vi "add points 2.0.vi"(10 "Spacing":dbl=1.0, 11 "Waypoints":dbl[][](array[numeric])) -> (3 "Path":dbl[][](array[numeric]) format="%#.3f")   [LabVIEW 2018]
panel:
  out "element":i32
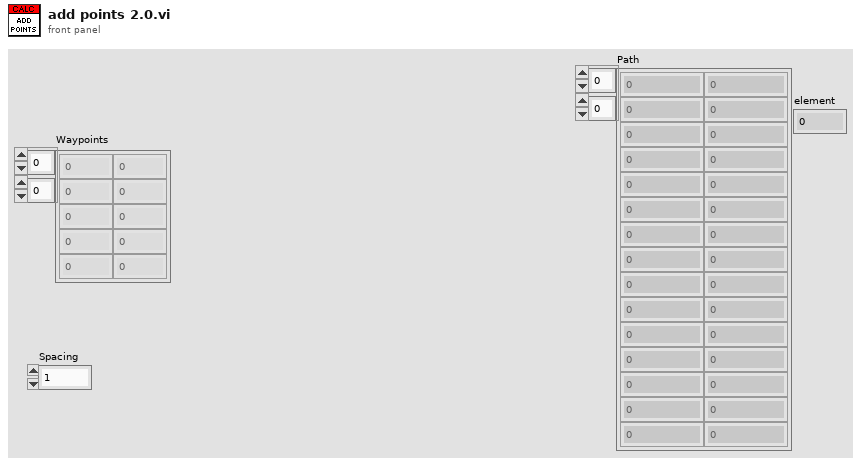
[diagram p1: front panel]
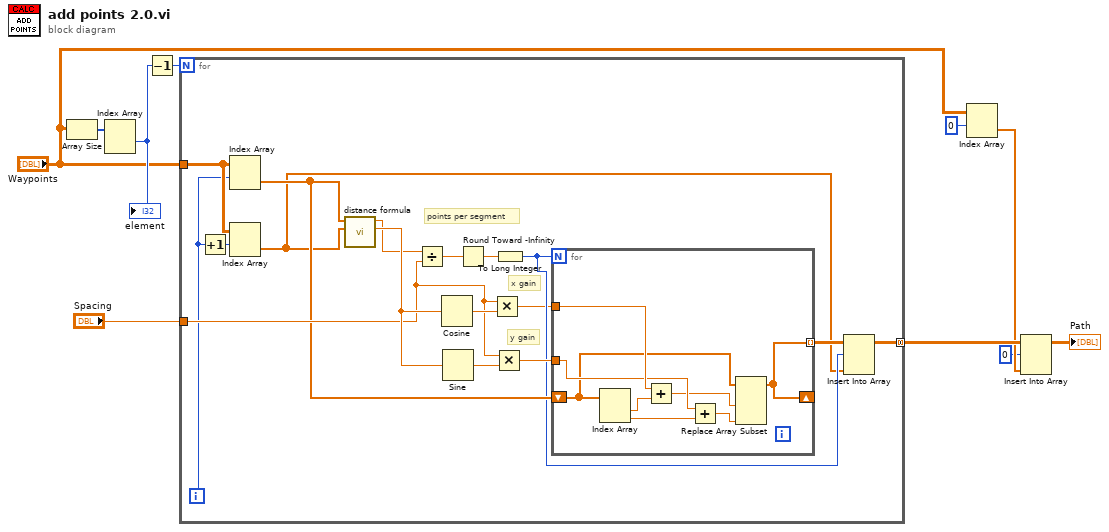
[diagram p0: block diagram]
diagram:
  n1 = Array Size(array="Waypoints") -> (size(s)=w10:i32[])
  n2 = Index Array(array=w10) -> (element #1=w9:i32)  [unwired: 2 in, 1 out]
  "element" <- w9
  n3 = Decrement(x=w9) -> (x-1=w6:i32)
  n4 = for {
    N: w6 -> [_]
    tunnel: "Waypoints" -> [w26]
    tunnel: "Spacing" -> [w20]
    tunnel: [w15] -> w7 mode=concatenating
    i -> [w16]
    # "y gain"
    # "x gain"
    # "points per segment"
    n5 = Increment(x=w16) -> (x+1=w27:i32)
    n6 = Index Array(array=w26, index (row)=w16) -> (element=w17:dbl[])  [unwired: 1 in]
    n7 = Index Array(array=w26, index (row)=w27) -> (element=w11:dbl[])  [unwired: 1 in]
    n8 = call "distance formula.vi"("Point Y"=w11, "Point X"=w17) -> ("Angle (rad)"=w23:dbl, "Distance"=w13:dbl)  [unwired: 8 in]
    n9 = Divide(x=w13, y=w20) -> (x/y=w25:dbl)
    n10 = Cosine(x=w23) -> (cos(x)=w22:dbl)
    n11 = Sine(x=w23) -> (sin(x)=w21:dbl)
    n12 = Round Toward -Infinity(1:w25) -> (0:w24:dbl)
    n13 = Multiply(x=w20, y=w22) -> (x*y=w12:dbl)
    n14 = Multiply(x=w20, y=w21) -> (x*y=w19:dbl)
    n15 = To Long Integer(number=w24) -> (32bit integer=w14:i32)
    n16 = for {
      N: w14 -> [_]
      shift-right: [w28] -> _
      shift-left: w17 -> [w31]
      tunnel: w12 -> [w34]
      tunnel: w19 -> [w32]
      tunnel: [w28] -> w18 mode=indexing
      n17 = Index Array(array=w31) -> (element #1=w35:dbl, element #2=w33:dbl)  [unwired: 2 in]
      n18 = Add(x=w34, y=w35) -> (x+y=w30:dbl)
      n19 = Add(x=w32, y=w33) -> (x+y=w29:dbl)
      n20 = Replace Array Subset(array=w31, new element #1=w30, new element #2=w29) -> (w28:dbl[])  [unwired: 2 in]
    }
    n21 = Insert Into Array(array=w18, index (row)=w14, new element=w11) -> (w15:dbl[][])  [unwired: 1 in]
  }
  n22 = Index Array(array="Waypoints", index (row)=0) -> (element=w2:dbl[])  [unwired: 1 in]
  n23 = Insert Into Array(array=w7, index (row)=0, new element=w2) -> (→"Path":dbl[][])  [unwired: 1 in]
